vi "EXA_cancelCallback_command_abortackcmd.vi"(8 "error in (no error)":errorcluster) -> (0 "error out":errorcluster, 3 "function return":i32)   [LabVIEW 2016, in "SALLV_EXA.lvlib"]
doc: "int EXA_shm_cancelCallback_command_abort_ackcmdLV();"
uses:
  SALLV_EXA.lvlib
  SALLV_EXA.so
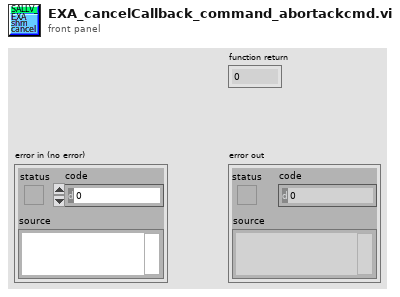
[diagram p1: front panel]
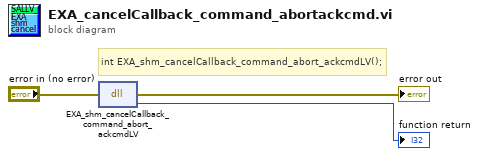
[diagram p0: block diagram]
diagram:
  # "int EXA_shm_cancelCallback_command_abort_ackcmdLV();"
  n1 = dll-call lib="home/hsundar/tcs/TEMP_EXA/SALLV_EXA.*" fn="EXA_shm_cancelCallback_command_abort_ackcmdLV"(error in="error in (no error)") -> (error out=→"error out":errorcluster, →"function return":i32)  [unwired: 2 in, 1 out]
